vi "Send I2C Transaction.vi"(8 "Error In":errorcluster, 10 "I2C Command":T1 {"Slave Address" format="%.0x"; "Register Address" format="%.0x"; "Data" format="%.0x"}, 11 "FPGA Ref in":refnum<k20>) -> (0 "Error Out":errorcluster, 2 "Read Data":u8 format="%.0x", 3 "FPGA Ref out":refnum<k20>)   [LabVIEW 2025, in "I2C Bus Monitor.lvclass"]
uses:
  I2C Bus Monitor.lvclass
  <instrlib>/FlexRIO/API/Host/v1/NI FlexRIO/API/Get Property Reference - Fpga Small.vi
  I2C Bus Monitor.lvclass/I2C Bus Monitor.ctl
  <instrlib>/FlexRIO/API/Host/v1/NI FlexRIO API v1.lvlib
  <resource>/objmgr/niflexrioapiChannel.rc
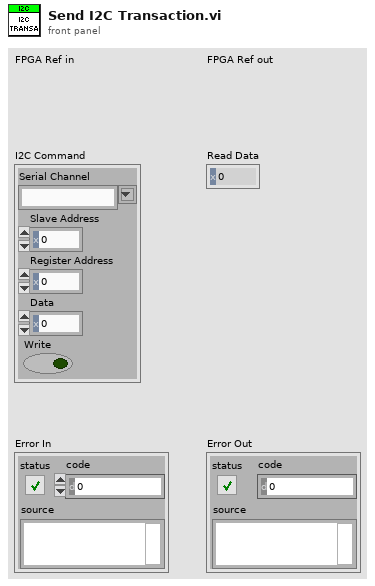
[diagram p1: front panel]
types:
  T1 = cluster{"Serial Channel":string, "Slave Address":u8, "Register Address":u16, "Data":u8, "Write":bool}
  T2 = enum16{"Serial Input Channel", "Serial Output Channel", "Unknown Channel Type"}
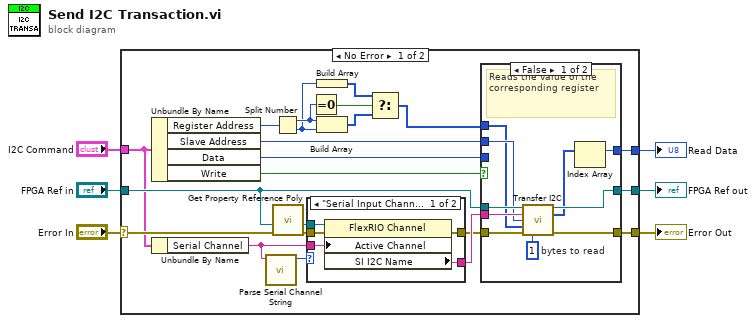
[diagram p0: block diagram]
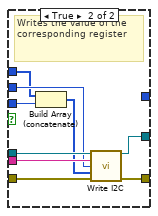
[diagram p2: hidden frame]
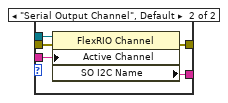
[diagram p3: hidden frame]
diagram:
  n1 = case shown="No Error" "Error In" {
    selector: "Error In" -> [w25 w58]
    tunnel: "FPGA Ref in" -> [w28 w59]
    tunnel: [w27 w59] -> w2
    tunnel: "I2C Command" -> [w9 _]
    tunnel: [w26 w58] -> w5
    tunnel: [w24 _] -> w1
    frame No Error {
      n2 = Unbundle By Name(w9) -> ("Register Address"=w23:u16, "Slave Address"=w7:u8, "Data"=w22:u8, "Write"=w8:bool)
      n3 = Unbundle By Name(w9) -> ("Serial Channel"=w16:string)
      n4 = call "Parse Serial Channel String.vi"("Serial Channel String"=w16) -> ("Serial Channel Type"=w21:T2)  [unwired: 9 in, 1 out]
      n5 = Split Number(x=w23) -> (hi(x)=w12:u8, lo(x)=w10:u8)
      n6 = call-poly <instrlib>:"Get Property Reference Poly.vi"("error in (no error)"=w25, "fpga interface in"=w28) -> ("error out"=w19:errorcluster, "property reference"=w20:refnum<k20>)  [unwired: 4 in, 1 out]
      n7 = case shown="\"Serial Input Channel\"" w21 {
        tunnel: [w52 w57] -> w18
        tunnel: [w51 w56] -> w17
        tunnel: w19 -> [w50 w55]
        tunnel: w20 -> [w49 w54]
        tunnel: w16 -> [w48 w53]
        frame "Serial Input Channel" {
          n8 = property class="FlexRIO Channel"(reference=w49, error in=w50, "Active Channel"=w48) -> (error out=w51:errorcluster, "SI I2C Name"=w52:string)  [unwired: 1 out]
        }
        frame "Serial Output Channel", Default {
          n9 = property class="FlexRIO Channel"(reference=w54, error in=w55, "Active Channel"=w53) -> (error out=w56:errorcluster, "SO I2C Name"=w57:string)  [unwired: 1 out]
        }
      }
      n10 = Equal To 0?(x=w12) -> (x = 0?=w13:bool)
      n11 = Build Array(w10) -> (w14:u8[])
      n12 = Build Array(w12, w10) -> (w15:u8[])
      n13 = Select(t=w14, s=w13, f=w15) -> (s? t:f=w11:u8[])
      n14 = case shown="False" w8 {
        tunnel: [w35 w43] -> w27
        tunnel: [w34 w42] -> w26
        tunnel: w28 -> [w38 w47]
        tunnel: w17 -> [w37 w46]
        tunnel: w18 -> [w36 w45]
        tunnel: w7 -> [w33 w40]
        tunnel: w22 -> [_ w41]
        tunnel: w11 -> [w32 w39]
        tunnel: [w30 _] -> w24
        frame False {
          w29 = u32 1  # bytes to read
          # "Reads the value of the corresponding register"
          n15 = call <instrlib>:"Transfer I2C.vi"("fpga interface in"=w38, "bus instance name"=w36, "slave address"=w33, "write data"=w32, "error in"=w37, "num bytes to read"=w29) -> ("fpga interface out"=w35:refnum<k20>, "read data"=w31:u8[], "error out"=w34:errorcluster)  [unwired: 6 in, 1 out]
          n16 = Index Array(array=w31) -> (element=w30:u8)  [unwired: 1 in]
        }
        frame True {
          # "Writes the value of the corresponding register"
          n17 = Build Array (concatenate)(w39, w41) -> (w44:u8[])
          n18 = call <instrlib>:"Write I2C.vi"("fpga interface in"=w47, "bus instance name"=w45, "slave address"=w40, "data"=w44, "error in"=w46) -> ("fpga interface out"=w43:refnum<k20>, "error out"=w42:errorcluster)  [unwired: 8 in, 1 out]
        }
      }
    }
    frame Error {
    }
  }
  "Error Out" <- w5
  "FPGA Ref out" <- w2
  "Read Data" <- w1
